vi "Abort Single Point Load-Ganging.vi"(8 "error in":errorcluster, 11 "Ganged Session In":T1) -> (0 "error out":errorcluster)   [LabVIEW 2021]
doc: "Abort the single point. In case of error resets the device for ganging configuration."
uses:
  controls/Abort Single Point-Ganging.ctl
  channel ganging/shared subVIs/ctl/NIDCPower_channel_ganging - ctl - ganged config.ctl
  channel ganging/shared subVIs/ctl/NIDCPower_channel_ganging - ctl - channel mode.ctl
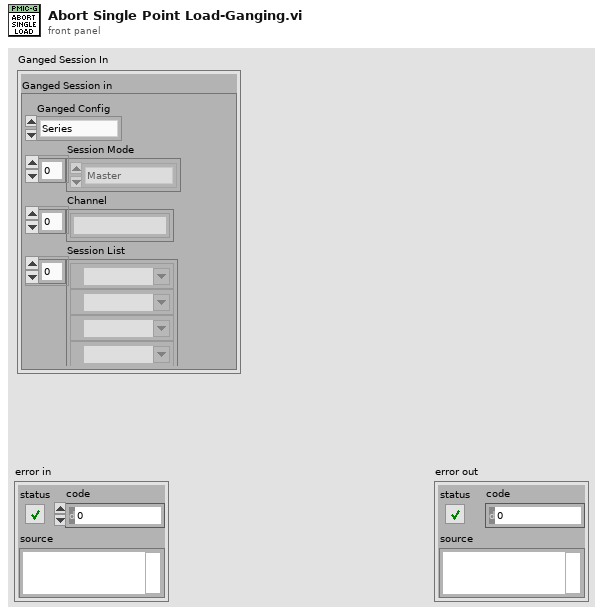
[diagram p1: front panel]
types:
  T1 = typedef "Abort Single Point-Ganging.ctl" = cluster{"Ganged Session in":cluster{"Ganged Config":T2, "Session List":refnum<k15>[], "Session Mode":T3[], "Channel":string[]}}
  T2 = typedef "NIDCPower_channel_ganging - ctl - ganged config.ctl" = enum32{"Series", "Parallel", "Manual"}
  T3 = typedef "NIDCPower_channel_ganging - ctl - channel mode.ctl" = enum32{"Master", "Slave", "Slave - Inverted"}
  T4 = cluster{"Ganged Config":T2, "Session List":refnum<k15>[], "Session Mode":T3[], "Channel":string[]}
  T5 = typedef "NIDCPower_channel_ganging - ctl - ganged session.ctl" = cluster{"Ganged Config":T2, "Session List":refnum<k15>[], "Session Mode":T3[], "Channel":string[]}
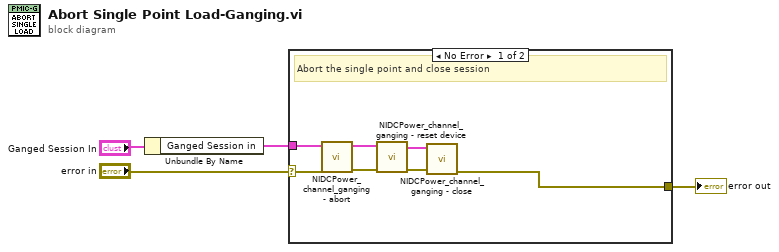
[diagram p0: block diagram]
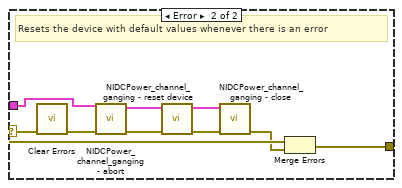
[diagram p2: hidden frame]
diagram:
  n1 = Unbundle By Name("Ganged Session In") -> ("Ganged Session in"=w1:T4)
  n2 = case shown="No Error" "error in" {
    selector: "error in" -> [w11 w14]
    tunnel: w1 -> [w9 w16]
    tunnel: [w10 w12] -> w3
    frame No Error {
      # "Abort the single point and close session"
      n3 = call "NIDCPower_channel_ganging - abort.vi"("error in (no error)"=w11, "Ganged Session In"=w9) -> ("error out"=w8:errorcluster, "Ganged Session Out"=w5:T5)  [unwired: 8 in]
      n4 = call "NIDCPower_channel_ganging - reset device.vi"("error in (no error)"=w8, "Ganged Session In"=w5) -> ("error out"=w7:errorcluster, "Ganged Session Out"=w6:T5)  [unwired: 8 in]
      n5 = call "NIDCPower_channel_ganging - close.vi"("error in (no error)"=w7, "Ganged Session In"=w6) -> ("error out"=w10:errorcluster)  [unwired: 9 in]
    }
    frame Error {
      # "Resets the device with default values whenever there is an error"
      n6 = call <vilib>:"Clear Errors.vi"("error in (no error)"=w14) -> ("error out"=w15:errorcluster)  [unwired: 5 in, 1 out]
      n7 = call "NIDCPower_channel_ganging - abort.vi"("error in (no error)"=w15, "Ganged Session In"=w16) -> ("error out"=w19:errorcluster, "Ganged Session Out"=w20:T5)  [unwired: 8 in]
      n8 = call "NIDCPower_channel_ganging - reset device.vi"("error in (no error)"=w19, "Ganged Session In"=w20) -> ("error out"=w17:errorcluster, "Ganged Session Out"=w18:T5)  [unwired: 8 in]
      n9 = call "NIDCPower_channel_ganging - close.vi"("error in (no error)"=w17, "Ganged Session In"=w18) -> ("error out"=w13:errorcluster)  [unwired: 9 in]
      n10 = Merge Errors(w14, w13) -> (w12:errorcluster)
    }
  }
  "error out" <- w3
